vi "SR430_set_bins_per_record.vi"(0 "address":T1, 2 "binsPerRecord":i32, 5 "error in (no error)":errorcluster) -> (14 "address out":T1, 19 "error out":errorcluster)   [LabVIEW 2015, in "SR430Driver.lvlib"]
doc: "Sets the bins per record of the SR430.\n\nThe \"bins per record\" can have the following values:\n1: 1024\n2: 2048\n...\n16: 16384\n\nCopyright (C)\nGesellschaft für Schwerionenforschung, GSI\nPlanckstr. 1\n64291 Darmstadt\nGermany\n\nContact: D.Beck@gsi.de \n\nThis program is free software; you can redistribute it and/or modify it under the terms of the \nGNU General Public License as published by the Free Software Foundation; either version 2 of the license, or (at your option) any later version.\n\nThis program is distributed in the hope that it will be useful, but WITHOUT ANY WARRANTY; without even the implied warranty of MERCHANTABILITY or FITNESS FOR A PARTICULAR PURPOSE. See the GNU General License for more details (http://www.gnu.org).\n\nGesellschaft für Schwerionenforschung, GSI\nPlanckstr. 1, 64291 Darmstadt, Germany\nFor all questions and ideas contact: M.Richter@gsi.de, K.Poppensieker, H.Brand@gsi.de or D.Beck@gsi.de.\nLast update: 11-APR-2002"
uses:
  SR430Driver.lvlib
  SR430_VISA Control.ctl
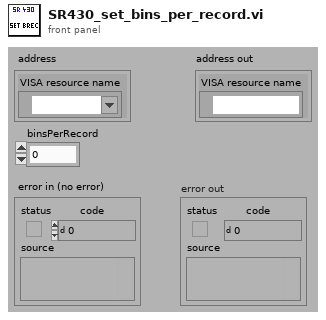
[diagram p1: front panel]
types:
  T1 = typedef "SR430Driver.lvlib/SR430_VISA Control.ctl" = cluster{"VISA resource name":refnum<visa-resource-name>}
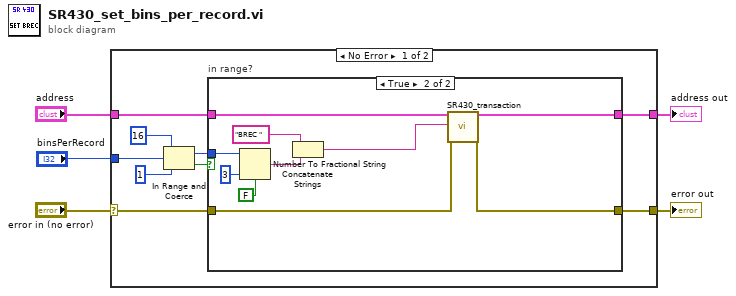
[diagram p0: block diagram]
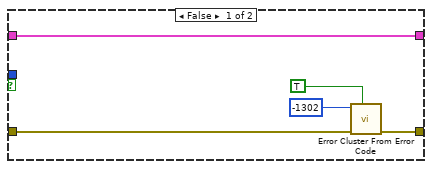
[diagram p2: hidden frame]
diagram:
  n1 = case shown="No Error" "error in (no error)" {
    selector: "error in (no error)" -> [w6 w30]
    tunnel: "address" -> [w14 w31]
    tunnel: [w13 w31] -> w4
    tunnel: [w12 w30] -> w3
    tunnel: "binsPerRecord" -> [w11 _]
    frame No Error {
      n2 = In Range and Coerce(upper limit=16, x=w11, lower limit=1) -> (coerced(x)=w7:i32, In Range?=w8:bool)
      n3 = case "in range?" shown="True" w8 {
        tunnel: w14 -> [w19 w25]
        tunnel: [w19 w24] -> w13
        tunnel: w6 -> [w18 w23]
        tunnel: [w17 w22] -> w12
        tunnel: w7 -> [_ w29]
        frame False {
          n4 = call <vilib>:"Error Cluster From Error Code.vi"("show call chain? (False)"=TRUE ("status"), "error in (no error)"=w18, "error code (0)"=-1302 ("code")) -> ("error out"=w17:errorcluster)  [unwired: 6 in]
        }
        frame True {
          n5 = Number To Fractional String(use system decimal point (T)=FALSE, number=w29, precision (6)=i16 3) -> (F-format string=w27:string)  [unwired: 1 in]
          n6 = Concatenate Strings("BREC ", w27) -> (w21:string)
          n7 = call "SR430_transaction.vi"("SR430 VISA Cluster"=w25, "SR430 Command String"=w21, "error in (no error)"=w23) -> ("dup SR430 VISA Cluster"=w24:T1, "error out"=w22:errorcluster)  [unwired: 13 in, 2 out]
        }
      }
    }
    frame Error {
    }
  }
  "address out" <- w4
  "error out" <- w3
